vi "GC copyright.vi"(2 "year":u16, 3 "code title":string) -> ()   [LabVIEW 2010]
panel:
  out "Info":string
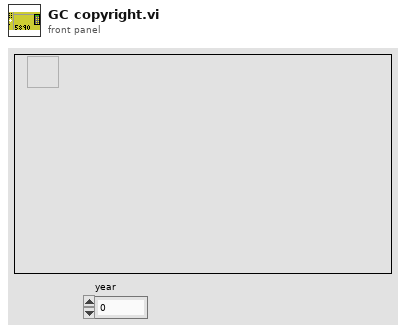
[diagram p1: front panel]
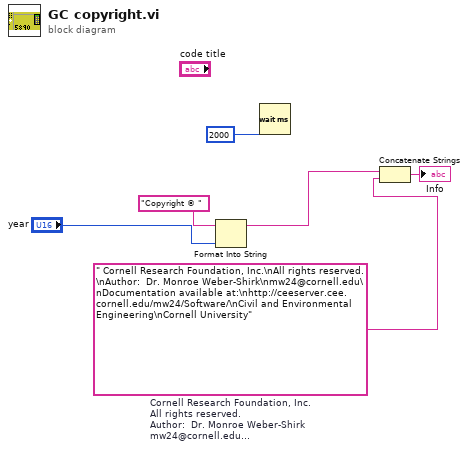
[diagram p0: block diagram]
diagram:
  w2 = " Cornell Research Foundation, Inc.\nAll rights reserved.\nAuthor:  Dr. Monroe Weber-Shirk\nmw24@cornell.edu\nDocumentation available at:\nhttp://ceeserver.cee.cornell.edu/mw24/Software/\nCivil and Environmental Engineering\nCornell University"  # Cornell Research Foundation, Inc. All rights reserved. Author:  Dr. Monroe Weber-Shirk mw24@cornell.edu Documentation available at: http://ceeserver.cee.cornell.edu/mw24/Software/ Civil and Environmental Engineering Cornell University
  n1 = Format Into String(initial string="Copyright © ", "year") -> (resulting string=w3:string)  [unwired: 2 in, 1 out]
  n2 = Wait (ms)(milliseconds to wait=2000) -> ()  [unwired: 1 out]
  n3 = Concatenate Strings(w3, w2) -> (→"Info":string)
